vi "Get FileMask.vi"(8 "error in (no error)":errorcluster, 11 "FileTransferOptions in":refnum<class "FileTransferOptions.lvclass">) -> (0 "error out":errorcluster, 2 "FileMask":string, 3 "FileTransferOptions out":refnum<class "FileTransferOptions.lvclass">)   [LabVIEW 2015, in "WinSCP.lvlib" / "FileTransferOptions.lvclass"]
uses:
  FileTransferOptions.lvclass
  FileTransferOptions.lvclass/FileTransferOptions.ctl
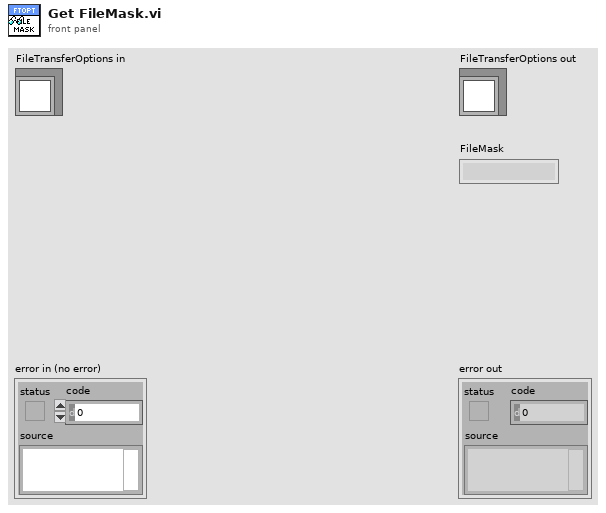
[diagram p1: front panel]
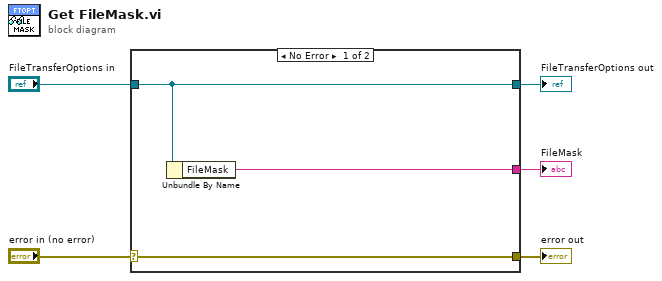
[diagram p0: block diagram]
diagram:
  n1 = case shown="No Error" "error in (no error)" {
    selector: "error in (no error)" -> [w8 w9]
    tunnel: [w8 w9] -> w4
    tunnel: [w7 w10] -> w2
    tunnel: "FileTransferOptions in" -> [w7 w10]
    tunnel: [w6 _] -> w1
    frame No Error {
      n2 = Unbundle By Name(w7) -> ("FileMask"=w6:string)
    }
    frame Error {
    }
  }
  "error out" <- w4
  "FileTransferOptions out" <- w2
  "FileMask" <- w1
